vi "Remove 2D Array Global Outliers (SGL) with Mask.vi"(6 "Init?":bool, 8 "Error In":errorcluster, 9 "2D Mask in":bool[][](array[boolean]), 11 "2D Array in":sgl[][](array[numeric])) -> (0 "Error Out":errorcluster, 2 "# Modified Values":i32, 3 "2D Array out":sgl[][](array[numeric]))   [LabVIEW 2021]
uses:
  6b6b94e1-32ac-4c5d-ae91-2d6312532ec6.vi/aaefba88-e7b4-4d4f-b2fa-6036c27193be.vi
  6b6b94e1-32ac-4c5d-ae91-2d6312532ec6.vi/aaefba88-e7b4-4d4f-b2fa-6036c27193be.vi/59314c09-68ff-4b78-8684-0242d4040ca4.vi
  6b6b94e1-32ac-4c5d-ae91-2d6312532ec6.vi/aaefba88-e7b4-4d4f-b2fa-6036c27193be.vi/59314c09-68ff-4b78-8684-0242d4040ca4.vi/d4db2432-cc9c-482c-8957-dac855435ef6.vi
  6b6b94e1-32ac-4c5d-ae91-2d6312532ec6.vi/aaefba88-e7b4-4d4f-b2fa-6036c27193be.vi/59314c09-68ff-4b78-8684-0242d4040ca4.vi/86fbf154-bd7b-49a2-8ab2-a837b2a95f24.vi
  6b6b94e1-32ac-4c5d-ae91-2d6312532ec6.vi/aaefba88-e7b4-4d4f-b2fa-6036c27193be.vi/59314c09-68ff-4b78-8684-0242d4040ca4.vi/3b95b01e-1ec2-4565-bcd9-7606a5281010.vi
  6b6b94e1-32ac-4c5d-ae91-2d6312532ec6.vi/aaefba88-e7b4-4d4f-b2fa-6036c27193be.vi/59314c09-68ff-4b78-8684-0242d4040ca4.vi/96a08935-737a-44b2-979c-a81d56408f7e.vi
  6b6b94e1-32ac-4c5d-ae91-2d6312532ec6.vi/aaefba88-e7b4-4d4f-b2fa-6036c27193be.vi/59314c09-68ff-4b78-8684-0242d4040ca4.vi/d4db2432-cc9c-482c-8957-dac855435ef6.vi/6eaecd13-6e48-4772-a921-b51ebdf84d88.vi
  6b6b94e1-32ac-4c5d-ae91-2d6312532ec6.vi/aaefba88-e7b4-4d4f-b2fa-6036c27193be.vi/59314c09-68ff-4b78-8684-0242d4040ca4.vi/d4db2432-cc9c-482c-8957-dac855435ef6.vi/d2d5f2b7-06f4-47f6-971c-049c3fdbb653.vi
  6b6b94e1-32ac-4c5d-ae91-2d6312532ec6.vi/aaefba88-e7b4-4d4f-b2fa-6036c27193be.vi/59314c09-68ff-4b78-8684-0242d4040ca4.vi/3b95b01e-1ec2-4565-bcd9-7606a5281010.vi/6eaecd13-6e48-4772-a921-b51ebdf84d88.vi
  6b6b94e1-32ac-4c5d-ae91-2d6312532ec6.vi/aaefba88-e7b4-4d4f-b2fa-6036c27193be.vi/59314c09-68ff-4b78-8684-0242d4040ca4.vi/3b95b01e-1ec2-4565-bcd9-7606a5281010.vi/d2d5f2b7-06f4-47f6-971c-049c3fdbb653.vi
  6b6b94e1-32ac-4c5d-ae91-2d6312532ec6.vi/aaefba88-e7b4-4d4f-b2fa-6036c27193be.vi/59314c09-68ff-4b78-8684-0242d4040ca4.vi/96a08935-737a-44b2-979c-a81d56408f7e.vi/6eaecd13-6e48-4772-a921-b51ebdf84d88.vi
  6b6b94e1-32ac-4c5d-ae91-2d6312532ec6.vi/aaefba88-e7b4-4d4f-b2fa-6036c27193be.vi/59314c09-68ff-4b78-8684-0242d4040ca4.vi/96a08935-737a-44b2-979c-a81d56408f7e.vi/d2d5f2b7-06f4-47f6-971c-049c3fdbb653.vi
  <vilib>/Utility/error.llb/Error Cluster From Error Code.vi
  <vilib>/ErrorRing/Error Ring.xnode
  <vilib>/Comparison/Less/Less Functor/Less Functor.lvclass
panel:
  out "CPU (s)":dbl
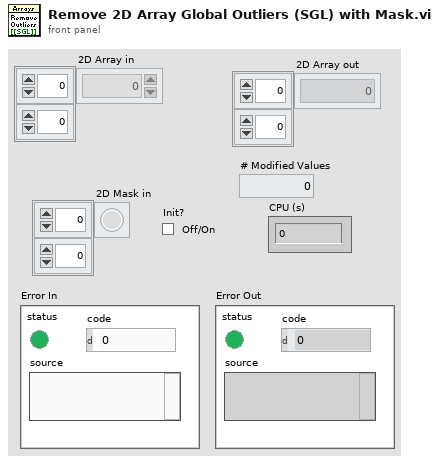
[diagram p1: front panel]
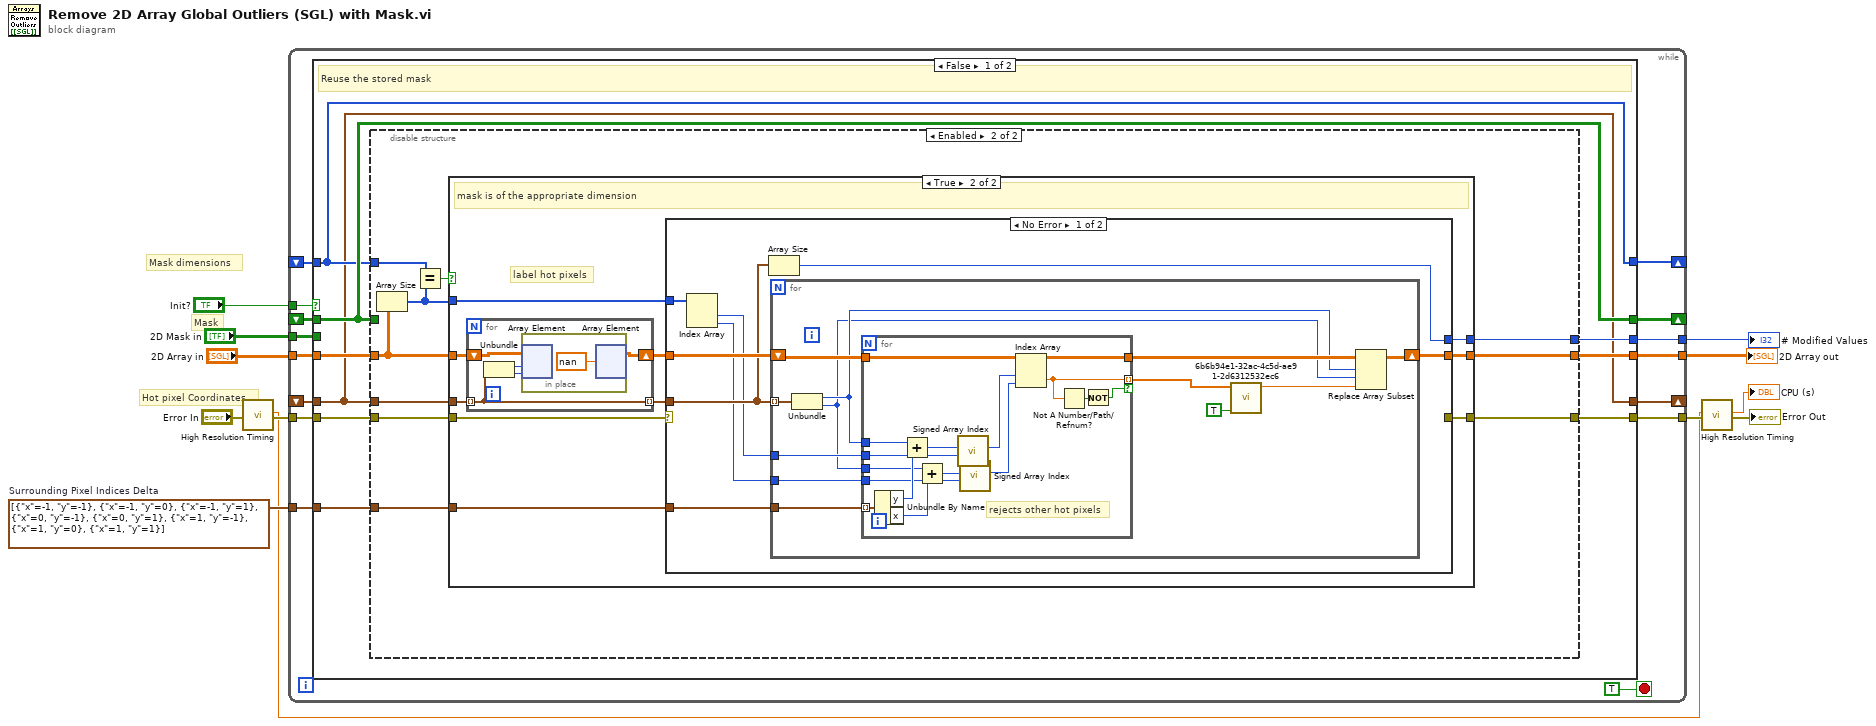
[diagram p0: block diagram]
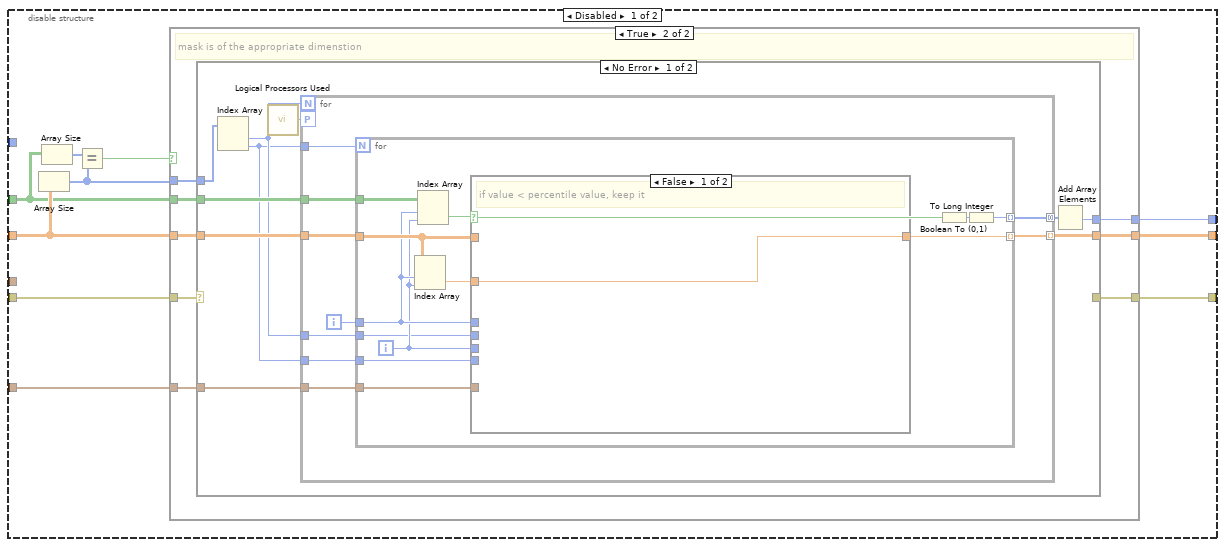
[diagram p2: hidden frame]
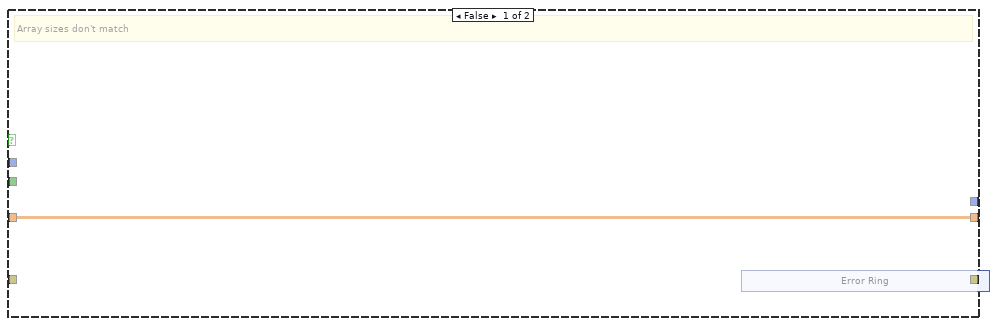
[diagram p3: hidden frame]
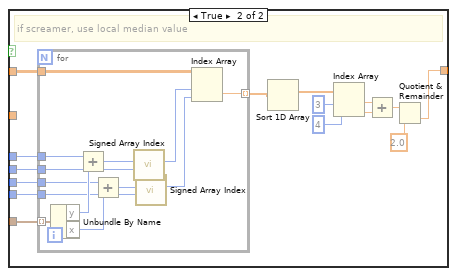
[diagram p4: hidden frame]
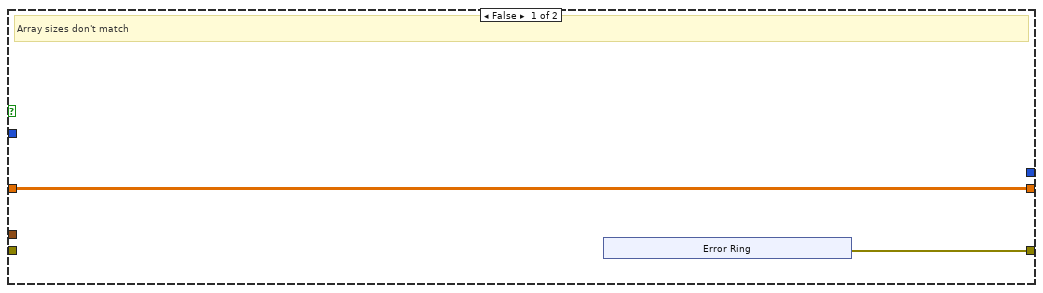
[diagram p6: hidden frame]
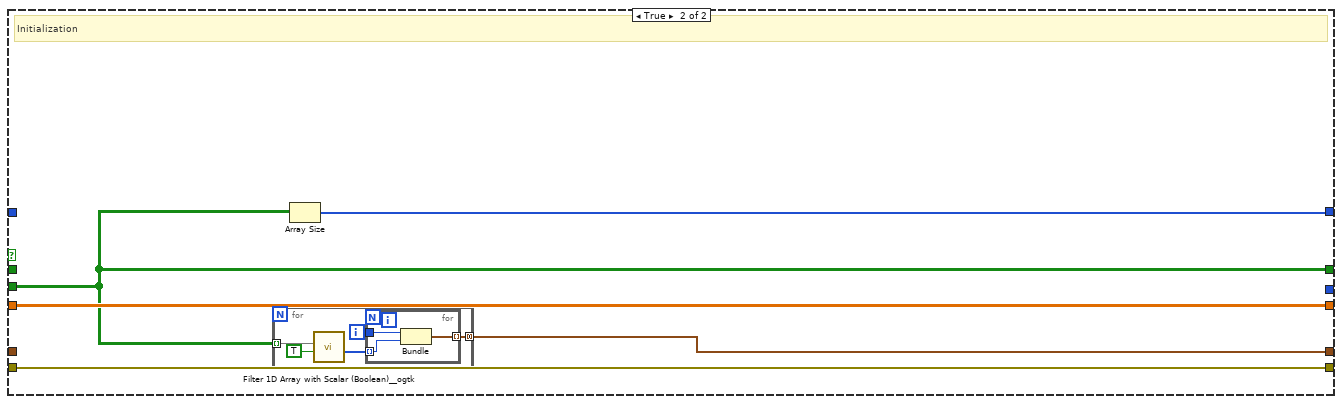
[diagram p8: hidden frame]
diagram:
  w11 = cluster{"x":i32, "y":i32}[] [{"x"=-1, "y"=-1}, {"x"=-1, "y"=0}, {"x"=-1, "y"=1}, {"x"=0, "y"=-1}, {"x"=0, "y"=1}, {"x"=1, "y"=-1}, {"x"=1, "y"=0}, {"x"=1, "y"=1}]  # Surrounding Pixel Indices Delta
  # "Mask"
  # "Hot pixel Coordinates"
  # "Mask dimensions"
  n1 = call "High Resolution Timing.vi"("Error In"="Error In") -> ("elapsed (relative) seconds"=w2:dbl, "Error Out"=w3:errorcluster)  [unwired: 16 in, 1 out]
  n2 = while {
    tunnel: w11 -> [w26]
    tunnel: [w22] -> w9
    tunnel: "Init?" -> [w21]
    tunnel: "2D Array in" -> [w27]
    tunnel: [w23] -> w10
    shift-right: [w19] -> _
    shift-left: _ -> [w17]
    tunnel: "2D Mask in" -> [w18]
    tunnel: w3 -> [w25]
    tunnel: [w24] -> w6
    shift-right: [w16] -> _
    shift-left: _ -> [w15]
    shift-right: [w14] -> _
    shift-left: _ -> [w13]
    stop <- TRUE stop-if-true
    n3 = case shown="False" w21 {
      tunnel: w27 -> [w36 w195]
      tunnel: w26 -> [w35 _]
      tunnel: w25 -> [w34 w196]
      tunnel: [w33 w196] -> w24
      tunnel: [w32 w195] -> w23
      tunnel: [w31 _] -> w22
      tunnel: [w30 w193] -> w19
      tunnel: w18 -> [_ w193]
      tunnel: w17 -> [w30 _]
      tunnel: [w28 w194] -> w16
      tunnel: w15 -> [w28 _]
      tunnel: [w29 w192] -> w14
      tunnel: w13 -> [w29 _]
      frame False {
        # "Reuse the stored mask"
        n4 = disable-structure shown="Enabled" {
          disable-tunnel: w36 -> [w46 w132]
          disable-tunnel: w35 -> [w45 w131]
          disable-tunnel: w34 -> [w44 w130]
          disable-tunnel: [w43 w129] -> w33
          disable-tunnel: [w42 w128] -> w32
          disable-tunnel: [w41 w127] -> w31
          disable-tunnel: w30 -> [w37 _]
          disable-tunnel: w29 -> [_ w124]
          disable-tunnel: w28 -> [_ w123]
          frame Disabled {
            n5 = Array Size(array=w46) -> (size(s)=w39:i32[])
            n6 = Array Size(array=w37) -> (size(s)=w40:i32[])
            n7 = Equal?(x=w40, y=w39) -> (x = y?=w38:bool)
            n8 = case shown="True" w38 {
              tunnel: w46 -> [w48 w60]
              tunnel: w45 -> [_ w59]
              tunnel: w44 -> [_ w58]
              tunnel: [w47 w57] -> w43
              tunnel: [w48 w56] -> w42
              tunnel: [_ w55] -> w41
              tunnel: w39 -> [_ w54]
              tunnel: w37 -> [_ w53]
              frame False {
                # "Array sizes don't match"
                n9 = xnode "Error Ring"() -> ("error out"=w47:errorcluster)
              }
              frame True {
                # "mask is of the appropriate dimenstion"
                n10 = case shown="No Error" w58 {
                  selector: w58 -> [_ w121]
                  tunnel: w59 -> [w70 _]
                  tunnel: [w69 w122] -> w56
                  tunnel: w60 -> [w68 w122]
                  tunnel: w54 -> [w67 _]
                  tunnel: [_ w121] -> w57
                  tunnel: [w63 _] -> w55
                  tunnel: w53 -> [w64 _]
                  frame No Error {
                    n11 = Index Array(array=w67) -> (element #1=w62:i32, element #2=w61:i32)  [unwired: 2 in]
                    n12 = call "Logical Processors Used.vi"() -> ("# Logical Processor Used"=w66:i32)  [unwired: 6 in]
                    n13 = for {
                      N: w62 -> [_]
                      tunnel: w68 -> [w79]
                      tunnel: w70 -> [w78]
                      tunnel: [w77] -> w69 mode=indexing
                      tunnel: w61 -> [w73]
                      workers-P: w66 -> [_]
                      tunnel: [w75] -> w65 mode=concatenating
                      tunnel: w64 -> [w74]
                      tunnel: w62 -> [w72]
                      tunnel: w61 -> [w71]
                      i -> [w76]
                      n14 = for {
                        N: w73 -> [_]
                        tunnel: w76 -> [w89]
                        tunnel: w79 -> [w90]
                        tunnel: w78 -> [w91]
                        tunnel: [w88] -> w77 mode=indexing
                        tunnel: [w85] -> w75 mode=indexing
                        tunnel: w74 -> [w84]
                        tunnel: w72 -> [w81]
                        tunnel: w71 -> [w80]
                        i -> [w83]
                        n15 = Index Array(array=w90, index (row)=w89, index (col)=w83) -> (element=w82:sgl)
                        n16 = Index Array(array=w84, index (row)=w89, index (col)=w83) -> (element=w87:bool)
                        n17 = case shown="False" w87 {
                          tunnel: w91 -> [_ w107]
                          tunnel: w90 -> [_ w100]
                          tunnel: w89 -> [_ w99]
                          tunnel: w83 -> [_ w98]
                          tunnel: [w92 w97] -> w88
                          tunnel: w82 -> [w92 _]
                          tunnel: w81 -> [_ w94]
                          tunnel: w80 -> [_ w93]
                          frame False {
                            # "if value < percentile value, keep it"
                          }
                          frame True {
                            # "if screamer, use local median value"
                            n18 = for {
                              tunnel: w100 -> [w115]
                              tunnel: w107 -> [w120] mode=indexing
                              tunnel: w99 -> [w119]
                              tunnel: w98 -> [w117]
                              tunnel: [w114] -> w96 mode=indexing
                              tunnel: w94 -> [w111]
                              tunnel: w93 -> [w108]
                              n19 = Unbundle By Name(w120) -> ("y"=w118:i32, "x"=w116:i32)
                              n20 = Add(x=w119, y=w118) -> (x+y=w113:i32)
                              n21 = Add(x=w117, y=w116) -> (x+y=w110:i32)
                              n22 = call "Signed Array Index.vi"("Array Size"=w111, "Array Index in"=w113) -> ("Array Index out"=w112:i32)  [unwired: 9 in]
                              n23 = call "Signed Array Index.vi"("Array Size"=w108, "Array Index in"=w110) -> ("Array Index out"=w109:i32)  [unwired: 9 in]
                              n24 = Index Array(array=w115, index (row)=w112, index (col)=w109) -> (element=w114:sgl)
                            }
                            n25 = Sort 1D Array(array=w96) -> (sorted array=w95:sgl[])
                            n26 = Index Array(array=w95, index #1=3 ("index"), index #2=4 ("index")) -> (element #1=w104:sgl, element #2=w103:sgl)
                            n27 = Add(x=w104, y=w103) -> (x+y=w102:sgl)
                            n28 = Quotient & Remainder(x=w102, y=sgl 2.0) -> (floor(x/y)=w97:sgl)  [unwired: 1 out]
                          }
                        }
                        n29 = Boolean To (0,1)(Boolean=w87) -> (0, 1=w86:i16)
                        n30 = To Long Integer(number=w86) -> (32bit integer=w85:i32)
                      }
                    }
                    n31 = Add Array Elements(numeric array=w65) -> (sum=w63:i32)
                  }
                  frame Error {
                  }
                }
              }
            }
          }
          frame Enabled {
            n32 = Array Size(array=w132) -> (size(s)=w126:i32[])
            n33 = Equal?(x=w124, y=w126) -> (x = y?=w125:bool)
            n34 = case shown="True" w125 {
              tunnel: w132 -> [w134 w140]
              tunnel: w131 -> [_ w148]
              tunnel: w130 -> [_ w147]
              tunnel: [w133 w146] -> w129
              tunnel: [w134 w145] -> w128
              tunnel: [_ w144] -> w127
              tunnel: w126 -> [_ w143]
              tunnel: w123 -> [_ w142]
              frame False {
                # "Array sizes don't match"
                n35 = xnode "Error Ring"() -> ("error out"=w133:errorcluster)
              }
              frame True {
                # "label hot pixels"
                # "mask is of the appropriate dimension"
                n36 = for {
                  tunnel: w142 -> [w152] mode=indexing
                  tunnel: [w152] -> w141 mode=indexing
                  shift-right: [w149] -> w139
                  shift-left: w140 -> [w153]
                  n37 = Unbundle(w152) -> (w150:i32, "Numeric"=w151:i32)
                  n38 = in-place {
                    n39 = in-place-array #1(w153, w150, w151) -> ()  [unwired: 1 out]
                    n40 = in-place-array #1(sgl nan ("element")) -> (w149:sgl[][])  [unwired: 2 out]
                  }
                }
                n41 = case shown="No Error" w147 {
                  selector: w147 -> [_ w190]
                  tunnel: w148 -> [w162 _]
                  tunnel: [w157 w191] -> w145
                  tunnel: w139 -> [w161 w191]
                  tunnel: w143 -> [w160 _]
                  tunnel: [_ w190] -> w146
                  tunnel: [w158 _] -> w144
                  tunnel: w141 -> [w159 _]
                  frame No Error {
                    n42 = Index Array(array=w160) -> (element #1=w156:i32, element #2=w155:i32)  [unwired: 2 in]
                    n43 = Array Size(array=w159) -> (size(s)=w158:i32)
                    n44 = for {
                      tunnel: w162 -> [w173]
                      tunnel: w156 -> [w172]
                      tunnel: w155 -> [w171]
                      tunnel: w159 -> [w170] mode=indexing
                      shift-right: [w167] -> w157
                      shift-left: w161 -> [w174]
                      n45 = Unbundle(w170) -> (w165:i32, "Numeric"=w164:i32)
                      n46 = for {
                        tunnel: w174 -> [w178]
                        tunnel: w173 -> [w189] mode=indexing
                        tunnel: w165 -> [w188]
                        tunnel: w164 -> [w186]
                        tunnel: [w175] -> w169 mode=indexing if=w176
                        tunnel: w172 -> [w182]
                        tunnel: w171 -> [w179]
                        tunnel: [w178] -> w168
                        # "rejects other hot pixels"
                        n47 = Unbundle By Name(w189) -> ("y"=w187:i32, "x"=w185:i32)
                        n48 = Add(x=w188, y=w187) -> (x+y=w184:i32)
                        n49 = Add(x=w186, y=w185) -> (x+y=w181:i32)
                        n50 = call "Signed Array Index.vi"("Array Size"=w182, "Array Index in"=w184) -> ("Array Index out"=w183:i32)  [unwired: 9 in]
                        n51 = call "Signed Array Index.vi"("Array Size"=w179, "Array Index in"=w181) -> ("Array Index out"=w180:i32)  [unwired: 9 in]
                        n52 = Index Array(array=w178, index (row)=w183, index (col)=w180) -> (element=w175:sgl)
                        n53 = Not A Number/Path/Refnum?(number/path/refnum=w175) -> (NaN/Path/Refnum?=w177:bool)
                        n54 = Not(x=w177) -> (.not. x?=w176:bool)
                      }
                      n55 = call "6b6b94e1-32ac-4c5d-ae91-2d6312532ec6.vi"("Reject NaN & +/- Inf (F)"=TRUE, "Array"=w169) -> ("Median"=w166:sgl)  [unwired: 9 in]
                      n56 = Replace Array Subset(array=w168, new element=w166, index (row)=w165, index (col)=w164) -> (w167:sgl[][])
                    }
                  }
                  frame Error {
                  }
                }
              }
            }
          }
        }
      }
      frame True {
        # "Initialization"
        n57 = for {
          tunnel: w193 -> [w201] mode=indexing
          tunnel: [w197] -> w194 mode=concatenating
          i -> [w198]
          n58 = call <userlib>:"Filter 1D Array with Scalar (Boolean)__ogtk.vi"("items to filter"=TRUE ("Boolean"), "array"=w201) -> ("filtered item indices"=w199:i32[])  [unwired: 4 in, 1 out]
          n59 = for {
            tunnel: w199 -> [w203] mode=indexing
            tunnel: w198 -> [w204]
            tunnel: [w202] -> w197 mode=indexing
            n60 = Bundle(w204, "Numeric"=w203) -> (w202:cluster{i32, "Numeric":i32})  [unwired: 1 in]
          }
        }
        n61 = Array Size(array=w193) -> (size(s)=w192:i32[])
      }
    }
  }
  "2D Array out" <- w10
  "# Modified Values" <- w9
  n62 = call "High Resolution Timing.vi"("relative seconds (NaN)"=w2, "Error In"=w6) -> ("elapsed (relative) seconds"=→"CPU (s)":dbl, "Error Out"=→"Error Out":errorcluster)  [unwired: 15 in, 1 out]
